vi "Reset uC.vi"(1 "TUBO":bool=TRUE, 2 "CUP":bool=TRUE, 3 "DEC":bool=TRUE, 4 "AH":bool=TRUE) -> ()   [LabVIEW 2018]
panel:
  # "ESTE VI ENVIA O COMANDO:\n\nPARA OS CONTROLADORES:"
  # "PROG RESET\n\nAH, DEC, CUP e TUBO"
  # "HABILITAR"
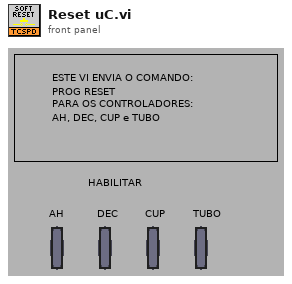
[diagram p1: front panel]
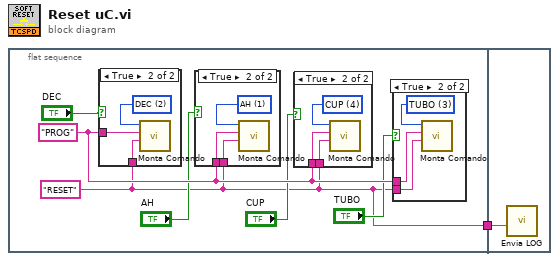
[diagram p0: block diagram]
diagram:
  n1 = flat-sequence {
    tunnel: [w2] -> w1
    tunnel: w1 -> [w20]
    frame #0 {
      w2 = "RESET" ("Comando")
      w7 = "PROG" ("Dispositivo")
      n2 = case shown="True" "DEC" {
        tunnel: w7 -> [_ w9]
        tunnel: w2 -> [_ w8]
        frame False {
        }
        frame True {
          w10 = u16 2 items=["ZERO", "AH", "DEC", "TUBO", "CUP"] ("Controlador")
          n3 = call "Monta Comando.vi"("Comando"=w8, "Dispositivo"=w9, "Controlador"=w10) -> ()  [unwired: 2 in, 5 out]
        }
      }
      n4 = case shown="True" "AH" {
        tunnel: w7 -> [_ w12]
        tunnel: w2 -> [_ w11]
        frame False {
        }
        frame True {
          w13 = u16 1 items=["ZERO", "AH", "DEC", "TUBO", "CUP"] ("Controlador")
          n5 = call "Monta Comando.vi"("Comando"=w11, "Dispositivo"=w12, "Controlador"=w13) -> ()  [unwired: 2 in, 5 out]
        }
      }
      n6 = case shown="True" "CUP" {
        tunnel: w7 -> [_ w15]
        tunnel: w2 -> [_ w14]
        frame False {
        }
        frame True {
          w16 = u16 4 items=["ZERO", "AH", "DEC", "TUBO", "CUP"] ("Controlador")
          n7 = call "Monta Comando.vi"("Comando"=w14, "Dispositivo"=w15, "Controlador"=w16) -> ()  [unwired: 2 in, 5 out]
        }
      }
      n8 = case shown="True" "TUBO" {
        tunnel: w7 -> [_ w18]
        tunnel: w2 -> [_ w17]
        frame False {
        }
        frame True {
          w19 = u16 3 items=["ZERO", "AH", "DEC", "TUBO", "CUP"] ("Controlador")
          n9 = call "Monta Comando.vi"("Comando"=w17, "Dispositivo"=w18, "Controlador"=w19) -> ()  [unwired: 2 in, 5 out]
        }
      }
    }
    frame #1 {
      n10 = call "Envia LOG.vi"("Comando a ser logado"=w20) -> ()  [unwired: 7 in, 2 out]
    }
  }
